vi "softWareBinCopyFTPMT2.vi"(8 "error in (no error)":errorcluster, 10 "RCNO":string, 11 "connection reference 2":T1) -> (0 "error out":errorcluster, 3 "connection reference":T1)   [LabVIEW 2012]
uses:
  <vilib>/addons/database/Connection.llb/Conn ObjectReference.ctl
  <vilib>/addons/database/Auxilliary.llb/DB Tools Cursor Type.ctl
  <vilib>/Utility/NIReport.llb/NI_report.lvclass
  <vilib>/addons/database/Connection.llb/Conn Execute.vi
  <vilib>/addons/database/Recordset.llb/Rec Fetch Recordset Data (R).vi
  <vilib>/Utility/NIReport.llb/Append Text Table to Report (wrap).vi
  <vilib>/addons/database/Recordset.llb/Rec Destroy - Connection.vi
  <vilib>/addons/database/_DB Variant To Data/Database Variant To Data.xnode
  <vilib>/addons/database/NI_Database_API.lvlib
  <vilib>/Utility/NIReport.llb/Excel/NI_Excel.lvclass
panel:
  out "error out 2":errorcluster
  out "Row Headers":string[](array[string])
  in  "Report Template":path=path "O:/Monitor/Report/MSTsoftBin.xls"
  out "concatenated string":string
  out "appended array":string[](array[string])
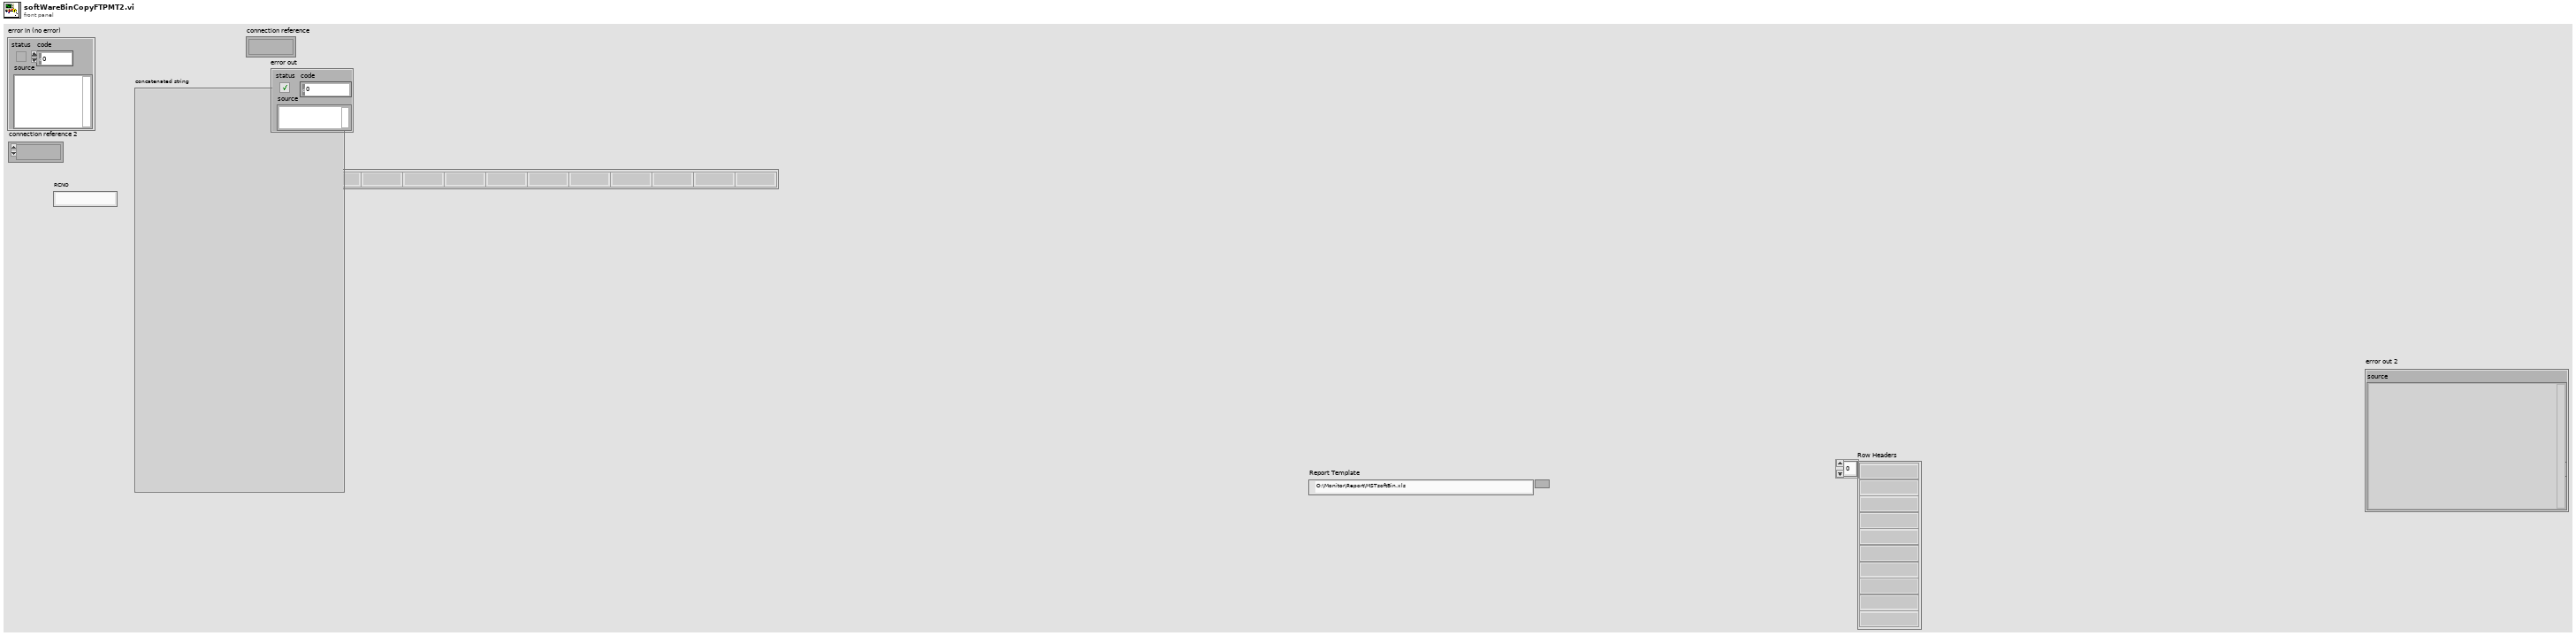
[diagram p1: front panel]
types:
  T1 = typedef "NI_Database_API.lvlib/Conn ObjectReference.ctl" = refnum<k1>
  T2 = enum16{"Standard Report", "HTML", "Word", "Excel"}
  T3 = typedef "NI_Database_API.lvlib/DB Tools Cursor Type.ctl" = enum16{"forward-only", "keyset", "dynamic", "static"}
  T4 = typedef "NI_Database_API.lvlib/Rec ObjectReference.ctl" = refnum<k1>
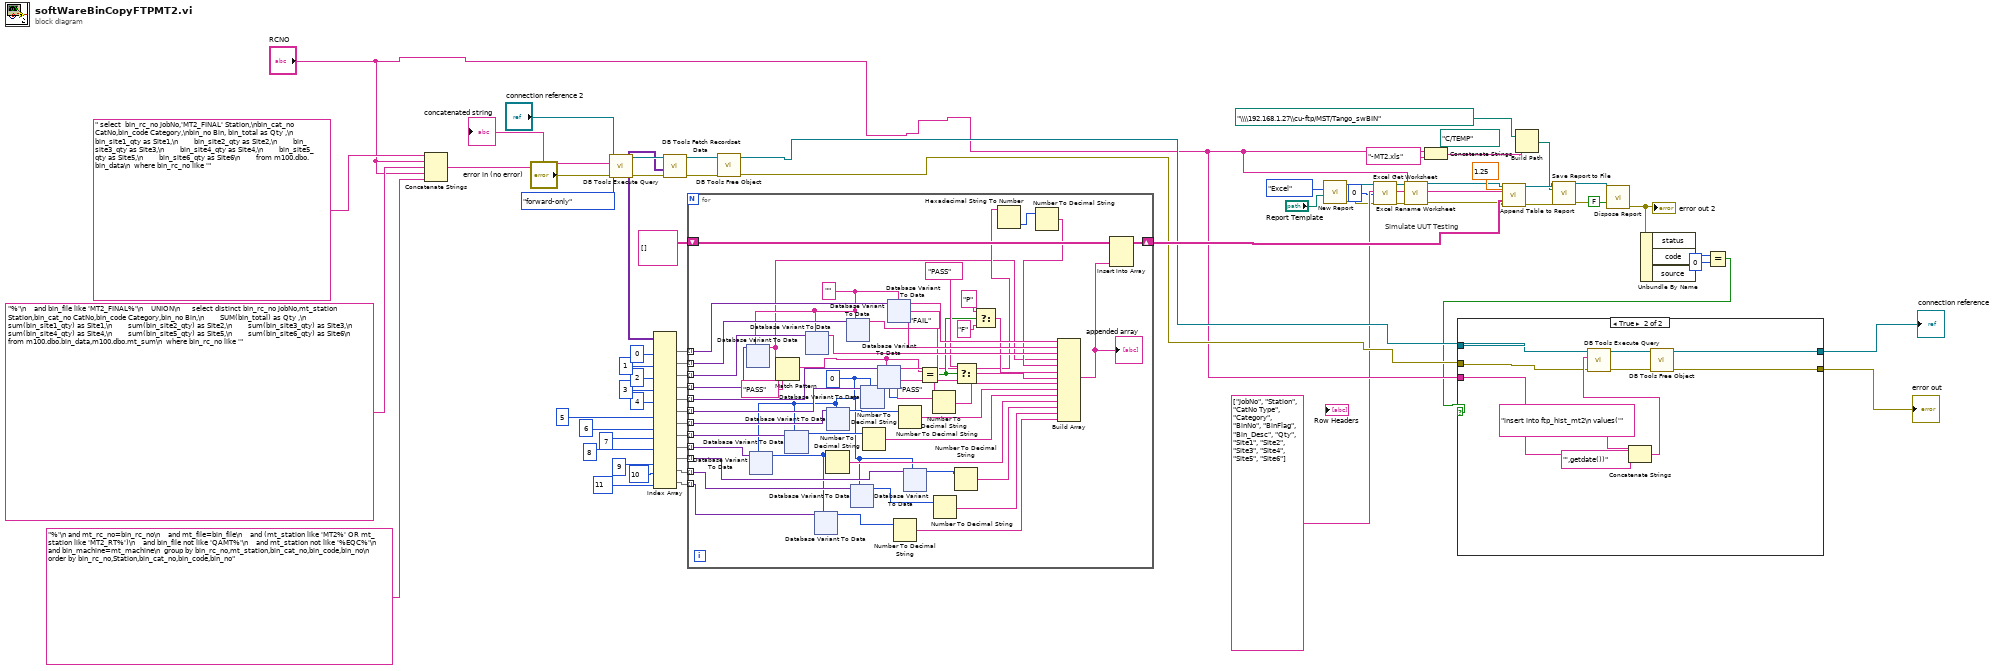
[diagram p0: block diagram]
diagram:
  (unwired) path "C:/TEMP" ("base path")
  # "Simulate UUT Testing"
  n1 = Concatenate Strings(" select  bin_rc_no JobNo,'MT2_FINAL' Station,\nbin_cat_no CatNo,bin_code Category,\nbin_no Bin, bin_total as Qty ,\n        bin_site1_qty as Site1,\n        bin_site2_qty as Site2,\n        bin_site3_qty as Site3,\n        bin_site4_qty as Site4,\n        bin_site5_qty as Site5,\n        bin_site6_qty as Site6\n        from m100.dbo.bin_data\n  where bin_rc_no like '" ("string"), "RCNO", "%'\n    and bin_file like 'MT2_FINAL%'\n    UNION\n      select distinct bin_rc_no JobNo,mt_station Station,bin_cat_no CatNo,bin_code Category,bin_no Bin,\n        SUM(bin_total) as Qty ,\n        sum(bin_site1_qty) as Site1,\n        sum(bin_site2_qty) as Site2,\n        sum(bin_site3_qty) as Site3,\n        sum(bin_site4_qty) as Site4,\n        sum(bin_site5_qty) as Site5,\n        sum(bin_site6_qty) as Site6\n        from m100.dbo.bin_data,m100.dbo.mt_sum\n  where bin_rc_no like '" ("string"), "RCNO", "%'\n and mt_rc_no=bin_rc_no\n    and mt_file=bin_file\n    and (mt_station like 'MT2%' OR mt_station like 'MT2_RT%')\n    and bin_file not like 'QAMT%'\n    and mt_station not like '%EQC%'\n    and bin_machine=mt_machine\n  group by bin_rc_no,mt_station,bin_cat_no,bin_code,bin_no\n  order by bin_rc_no,Station,bin_cat_no,bin_code,bin_no" ("string")) -> (w60:string)
  "concatenated string" <- w60
  n2 = call-poly <vilib>:"DB Tools Execute Query.vi"("error in (no error)"="error in (no error)", "cursor type"=DB_Tools_Cursor_Type."forward-only", "SQL query"=w60, "connection reference"="connection reference 2") -> ("error out"=w65:errorcluster, "recordset reference"=w67:T4)  [unwired: 4 in]
  n3 = call-poly <vilib>:"DB Tools Fetch Recordset Data.vi"("error in (no error)"=w65, "recordset reference"=w67) -> ("error out"=w64:errorcluster, "recordset data"=w59:variant[][], "recordset reference out"=w66:T4)  [unwired: 3 in]
  n4 = Index Array(array=w59, index (col) #1=0 ("disabled index (col)"), index (col) #2=1 ("index (col)"), index (col) #3=2 ("index (col)"), index (col) #4=3 ("index (col)"), index (col) #5=4 ("index (col)"), index (col) #6=5 ("index (col)"), index (col) #7=6 ("index (col)"), index (col) #8=7 ("index (col)"), index (col) #9=8 ("index (col)"), index (col) #10=9 ("index (col)"), index (col) #11=10 ("index (col)"), index (col) #12=11 ("index (col)")) -> (element #1=w48:variant[], element #2=w47:variant[], element #3=w46:variant[], element #4=w45:variant[], element #5=w44:variant[], element #6=w43:variant[], element #7=w42:variant[], element #8=w41:variant[], element #9=w40:variant[], element #10=w39:variant[], element #11=w36:variant[], element #12=w35:variant[])  [unwired: 12 in]
  n5 = for {
    tunnel: w48 -> [w115] mode=indexing
    tunnel: w47 -> [w114] mode=indexing
    tunnel: w46 -> [w113] mode=indexing
    tunnel: w45 -> [w112] mode=indexing
    tunnel: w44 -> [w111] mode=indexing
    tunnel: w43 -> [w110] mode=indexing
    tunnel: w42 -> [w109] mode=indexing
    tunnel: w41 -> [w108] mode=indexing
    tunnel: w40 -> [w107] mode=indexing
    tunnel: w39 -> [w106] mode=indexing
    tunnel: w36 -> [w97] mode=indexing
    tunnel: w35 -> [w96] mode=indexing
    shift-right: [w91] -> w33
    shift-left: string[][] [] ("array") -> [w90]
    w82 = 0
    w105 = ""
    n6 = xnode "Database Variant To Data"("database variant"=w112, "type"=w105) -> ("data"=w70:string)  [unwired: 1 in, 1 out]
    n7 = xnode "Database Variant To Data"("database variant"=w107, "type"=w82) -> ("data"=w94:i32)  [unwired: 1 in, 1 out]
    n8 = Match Pattern(string=w70, regular expression="PASS") -> (match substring=w68:string)  [unwired: 1 in, 3 out]
    n9 = xnode "Database Variant To Data"("database variant"=w108, "type"=w82) -> ("data"=w99:i32)  [unwired: 1 in, 1 out]
    n10 = xnode "Database Variant To Data"("database variant"=w113, "type"=w105) -> ("data"=w102:string)  [unwired: 1 in, 1 out]
    n11 = xnode "Database Variant To Data"("database variant"=w96, "type"=w94) -> ("data"=w95:i32)  [unwired: 1 in, 1 out]
    n12 = Number To Decimal String(number=w94) -> (decimal integer string=w86:string)  [unwired: 1 in]
    n13 = xnode "Database Variant To Data"("database variant"=w109, "type"=w82) -> ("data"=w100:i32)  [unwired: 1 in, 1 out]
    n14 = xnode "Database Variant To Data"("database variant"=w114, "type"=w105) -> ("data"=w103:string)  [unwired: 1 in, 1 out]
    n15 = xnode "Database Variant To Data"("database variant"=w97, "type"=w82) -> ("data"=w93:i32)  [unwired: 1 in, 1 out]
    n16 = xnode "Database Variant To Data"("database variant"=w110, "type"=w82) -> ("data"=w101:i32)  [unwired: 1 in, 1 out]
    n17 = Number To Decimal String(number=w99) -> (decimal integer string=w85:string)  [unwired: 1 in]
    n18 = xnode "Database Variant To Data"("database variant"=w111, "type"=w68) -> ("data"=w72:string)  [unwired: 1 in, 1 out]
    n19 = xnode "Database Variant To Data"("database variant"=w115, "type"=w105) -> ("data"=w104:string)  [unwired: 1 in, 1 out]
    n20 = Number To Decimal String(number=w95) -> (decimal integer string=w89:string)  [unwired: 1 in]
    n21 = Number To Decimal String(number=w100) -> (decimal integer string=w84:string)  [unwired: 1 in]
    n22 = xnode "Database Variant To Data"("database variant"=w106, "type"=w82) -> ("data"=w98:i32)  [unwired: 1 in, 1 out]
    n23 = Equal?(x=w68, y="PASS") -> (x = y?=w78:bool)
    n24 = Number To Decimal String(number=w101) -> (decimal integer string=w83:string)  [unwired: 1 in]
    n25 = Number To Decimal String(number=w93) -> (decimal integer string=w88:string)  [unwired: 1 in]
    n26 = Number To Decimal String(number=w98) -> (decimal integer string=w87:string)  [unwired: 1 in]
    n27 = Select(t="PASS", s=w78, f="FAIL") -> (s? t:f=w79:string)
    n28 = Select(t="P", s=w78, f="F") -> (s? t:f=w75:string)
    n29 = Hexadecimal String To Number(string=w72) -> (number=w73:u32)  [unwired: 2 in, 1 out]
    n30 = Number To Decimal String(number=w73) -> (decimal integer string=w71:string)  [unwired: 1 in]
    n31 = Build Array(w104, w103, w102, w70, w71, w75, w79, w83, w84, w85, w86, w87, w88, w89) -> (w92:string[])
    "appended array" <- w92
    n32 = Insert Into Array(array=w90, new element=w92) -> (w91:string[][])  [unwired: 2 in]
  }
  n33 = call-poly <vilib>:"DB Tools Free Object.vi"("error in (no error)"=w64, "recordset reference"=w66) -> ("error out"=w30:errorcluster, "connection reference"=w31:T1)  [unwired: 8 in]
  n34 = call <vilib>:"New Report.vi"("report type"=T2."Excel" ("Report Type"), "template (empty)"="Report Template") -> ("report out"=w24:refnum<class "NI_report.lvclass">, "error out"=w23:errorcluster)  [unwired: 12 in]
  n35 = call <vilib>:"Excel Get Worksheet.vi"("report in"=w24, "worksheet index (0)"=0, "error in (no error)"=w23) -> ("report out"=w21:refnum<class "NI_report.lvclass">, "error out"=w19:errorcluster)  [unwired: 11 in]
  n36 = call <vilib>:"Excel Rename Worksheet.vi"("report in"=w21, "worksheet name (\"\")"="RCNO", "error in (no error)"=w19) -> ("report out"=w20:refnum<class "NI_report.lvclass">, "error out"=w18:errorcluster)  [unwired: 11 in]
  n37 = Concatenate Strings("RCNO", "-MT2.xls" ("string")) -> (w11:string)
  n38 = call-poly <vilib>:"Append Table to Report.vi"("report in"=w20, "column width (1)"=1.25, "column headers"=string[] ["JobNo", "Station", "CatNo Type", "Category", "BinNo", "BinFlag", "Bin_Desc", "Qty", "Site1", "Site2", "Site3", "Site4", "Site5", "Site6"] ("row headers"), "text data"=w33, "error in (no error)"=w18) -> ("report out"=w14:refnum<class "NI_report.lvclass">, "error out"=w13:errorcluster)  [unwired: 7 in, 2 out]
  n39 = Build Path(base path=path "\\\\192.168.1.27\\cu-ftp/MST/Tango_swBIN", name or relative path=w11) -> (appended path=w10:path)
  n40 = call-dynamic "Save Report to File.vi"("report in"=w14, "report file path"=w10, "error in (no error)"=w13) -> ("report out"=w16:refnum<class "NI_report.lvclass">, "error out"=w15:errorcluster)  [unwired: 11 in]
  n41 = call-dynamic "Dispose Report.vi"("report in"=w16, "save changes? (F)"=FALSE, "error in (no error)"=w15) -> ("error out"=w9:errorcluster)  [unwired: 12 in]
  "error out 2" <- w9
  n42 = Unbundle By Name(w9) -> ("code"=w8:i32)  [unwired: 2 out]
  n43 = Equal?(x=w8, y=0) -> (x = y?=w6:bool)
  n44 = case shown="True" w6 {
    tunnel: w31 -> [w501 w511]
    tunnel: "RCNO" -> [_ w509]
    tunnel: [w501 w504] -> w5
    tunnel: [w500 w503] -> w4
    tunnel: w30 -> [w500 w502]
    frame False {
    }
    frame True {
      n45 = Concatenate Strings("insert into ftp_hist_mt2\n values('" ("string"), w509, "',getdate())" ("string")) -> (w507:string)
      n46 = call-poly <vilib>:"DB Tools Execute Query.vi"("error in (no error)"=w502, "SQL query"=w507, "connection reference"=w511) -> ("error out"=w505:errorcluster, "recordset reference"=w506:T4)  [unwired: 5 in]
      n47 = call-poly <vilib>:"DB Tools Free Object.vi"("error in (no error)"=w505, "recordset reference"=w506) -> ("error out"=w503:errorcluster, "connection reference"=w504:T1)  [unwired: 8 in]
    }
  }
  "connection reference" <- w5
  "error out" <- w4
